vi "sub_reduction_of_C.vi"(9 "dimension size":i32, 10 "L":sgl[](array[numeric]), 11 "K":dbl[][](array[numeric])) -> (3 "Real 2D Array":dbl[][](array[numeric]))   [LabVIEW 2019]
uses:
  <vilib>/Analysis/baseanly.llb/Real Inverse Matrix.vi
  <vilib>/Analysis/Matrix/Numeric/Multiply/Multiply - RM,RM.vi
  <vilib>/Analysis/Matrix/Numeric/Add/Add - RM,RM.vi
  <vilib>/Analysis/Matrix/Numeric/Conversions/Matrix To Array - RM.vi
  <vilib>/Analysis/NI_AALBase.lvlib
  <vilib>/Analysis/Matrix/NI_Matrix.lvlib
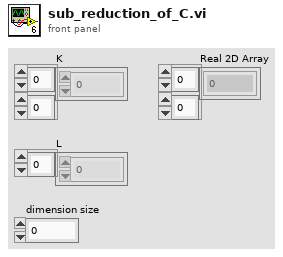
[diagram p1: front panel]
types:
  T1 = typedef "NI_Matrix.lvlib/RealMatrix.ctl" = dbl[][]
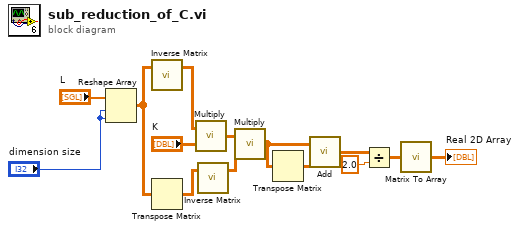
[diagram p0: block diagram]
diagram:
  n1 = Reshape Array("L", "dimension size", "dimension size") -> (w9:sgl[][])
  n2 = call-poly <vilib>:"Inverse Matrix.vi"("Input Matrix"=w9) -> ("Inverse Matrix"=w1:T1)  [unwired: 1 in, 1 out]
  n3 = Transpose Matrix(1:w9) -> (0:w7:dbl[][])
  n4 = call-poly <vilib>:"Multiply.vi"("Real Matrix B"="K", "Real Matrix A"=w1) -> ("A * B"=w3:T1)
  n5 = call-poly <vilib>:"Inverse Matrix.vi"("Input Matrix"=w7) -> ("Inverse Matrix"=w2:T1)  [unwired: 1 in, 1 out]
  n6 = call-poly <vilib>:"Multiply.vi"("Real Matrix B"=w2, "Real Matrix A"=w3) -> ("A * B"=w4:T1)
  n7 = Transpose Matrix(1:w4) -> (0:w5:T1)
  n8 = call-poly <vilib>:"Add.vi"("Real Matrix B"=w5, "Real Matrix A"=w4) -> ("A + B"=w6:T1)
  n9 = Divide(x=w6, y=2.0) -> (x/y=w10:T1)
  n10 = call-poly <vilib>:"Matrix To Array.vi"("Real Matrix"=w10) -> ("Real 2D Array"=→"Real 2D Array":dbl[][])
